vi "gantry移動定位.vi"() -> ()   [LabVIEW 2016]
uses:
  Classes/Controller/Motion/A3200 Folder/A3200.lvclass
panel:
  out "subarray":dbl[](array[numeric])
  in  "輸入定位":dbl[][](array[numeric])=[[200.0, 300.0]]
  out "Final Position":dbl[](array[numeric])
  out "Initial position":dbl[](array[numeric])
  in  "Speed (mm/s)":dbl=40.0
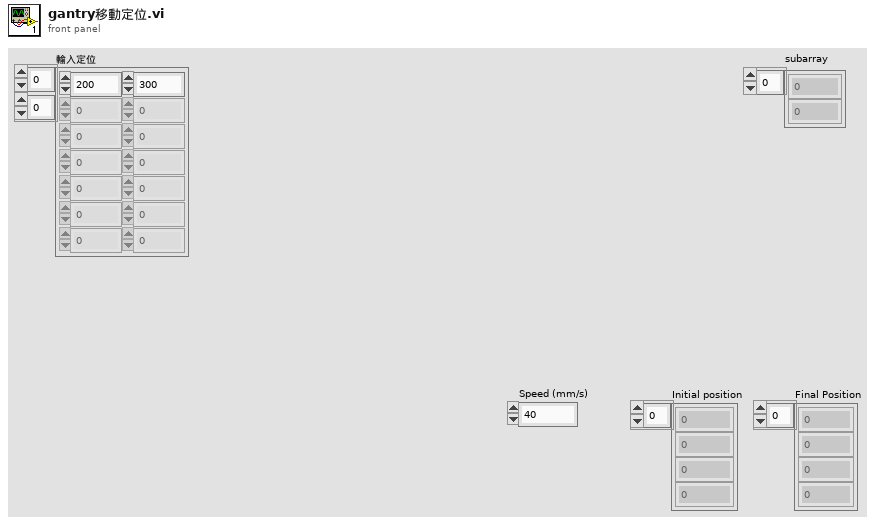
[diagram p1: front panel]
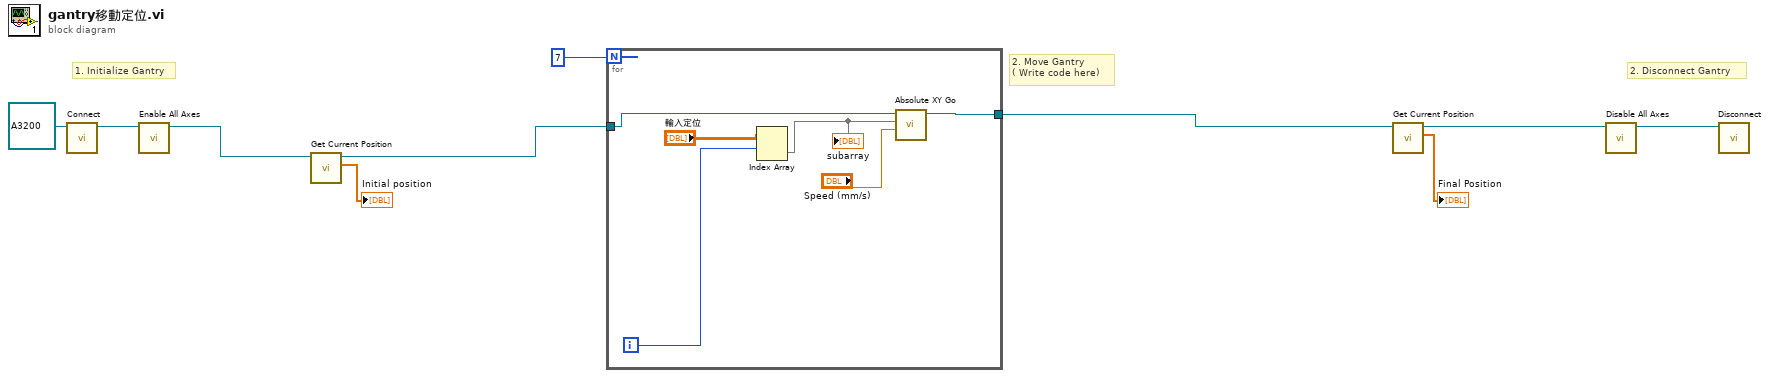
[diagram p0: block diagram]
diagram:
  # "1. Initialize Gantry"
  # "2. Disconnect Gantry"
  # "2. Move Gantry \n( Write code here)"
  n1 = call-dynamic "Connect.vi"("Gantry in"=refnum<class "A3200.lvclass"> refnum ("A3200.lvclass")) -> ("Gantry out"=w5:refnum<class "A3200.lvclass">)  [unwired: 9 in, 1 out]
  n2 = call-dynamic "Enable All Axes.vi"("A3200 in"=w5) -> ("A3200 out"=w4:refnum<class "A3200.lvclass">)  [unwired: 9 in, 1 out]
  n3 = call-dynamic "Get Current Position.vi"("Gantry in"=w4) -> ("XYZTheta Out"=→"Initial position":dbl[], "Gantry out"=w3:refnum<class "A3200.lvclass">)  [unwired: 8 in, 1 out]
  n4 = for {
    N: 7 -> [_]
    tunnel: w3 -> [w13]
    tunnel: [w12] -> w2
    i -> [w15]
    n5 = Index Array(array="輸入定位", index (row)=w15) -> (element=w11:dbl[])  [unwired: 1 in]
    "subarray" <- w11
    n6 = call-dynamic "Absolute XY Go.vi"("Speed"="Speed (mm/s)", "XY"=w11, "Gantry in"=w13) -> ("Gantry out"=w12:refnum<class "A3200.lvclass">)  [unwired: 7 in, 1 out]
  }
  n7 = call-dynamic "Get Current Position.vi"("Gantry in"=w2) -> ("XYZTheta Out"=→"Final Position":dbl[], "Gantry out"=w8:refnum<class "A3200.lvclass">)  [unwired: 8 in, 1 out]
  n8 = call-dynamic "Disable All Axes.vi"("Gantry in"=w8) -> ("Gantry out"=w9:refnum<class "A3200.lvclass">)  [unwired: 9 in, 1 out]
  n9 = call-dynamic "Disconnect.vi"("Gantry in"=w9) -> ()  [unwired: 9 in, 1 out]
